vi "Actor Core.vi"(8 "error in":errorcluster, 11 "Configuration in":refnum<class "Configuration.lvclass">) -> (0 "error out":errorcluster, 3 "Actor out":refnum<class "Actor.lvclass">)   [LabVIEW 2016, in "Configuration.lvlib" / "Configuration.lvclass"]
doc: "(<B>Filename</B>: Actor Framework.lvlib:Actor.lvclass:Actor Core.vi)\n\nReceives messages to the actor, reacts to them, and initiates any error handling that may shut the actor down.\n\nDescendant classes may override this VI to append parallel tasks for the actor to complete while it handles messages. Overrides use the Call Parent Method node."
uses:
  <userlib>/Configuration Dialog Actor/Configuration.lvclass
  C:/Program Files (x86)/National Instruments/LabVIEW 2016/vi.lib/ActorFramework/Actor/Actor.lvclass
  <vilib>/ActorFramework/Actor/Actor.lvclass
  <userlib>/Configuration Dialog Actor/Methods/Config Actor Core UI Ref.ctl
  <userlib>/Configuration Dialog Actor/Configuration.lvclass/Configuration.ctl
  <vilib>/ActorFramework/Actor/Actor.lvclass/Actor.ctl
  <vilib>/ActorFramework/Message Enqueuer/Message Enqueuer.lvclass/Message Enqueuer.ctl
  <userlib>/Configuration Dialog Actor/Configuration Messages/Display New Configuration SubPanel Msg/Display New Configuration SubPanel Msg.lvclass/Display New Configuration SubPanel Msg.ctl
  <vilib>/ActorFramework/Message Enqueuer/Init from Existing Queue.vi
  <vilib>/ActorFramework/Message Enqueuer/Enqueue.vi
  <vilib>/ActorFramework/Stop Msg/Stop Msg.lvclass
  C:/Program Files (x86)/National Instruments/LabVIEW 2016/vi.lib/ActorFramework/Message/Message.lvclass
  <userlib>/Configuration Messages/Change Password Msg/Change Password Msg.lvclass
  <userlib>/Configuration Dialog Actor/Configuration Messages/Display New Configuration SubPanel Msg/Display New Configuration SubPanel Msg.lvclass
  <userlib>/Configuration Dialog Actor/Configuration Messages/Display Help for Selected Category Msg/Display Help for Highlighted Category Msg.lvclass
  <vilib>/ActorFramework/Message Priority Queue/Priority Enqueue.vi
  <vilib>/ActorFramework/Message Enqueuer/Message Enqueuer.lvclass
panel:
  in  "Categories":i32(listbox)
  out "Title":string
  in  "Help":bool
  in  "OK":bool
  in  "Cancel":bool
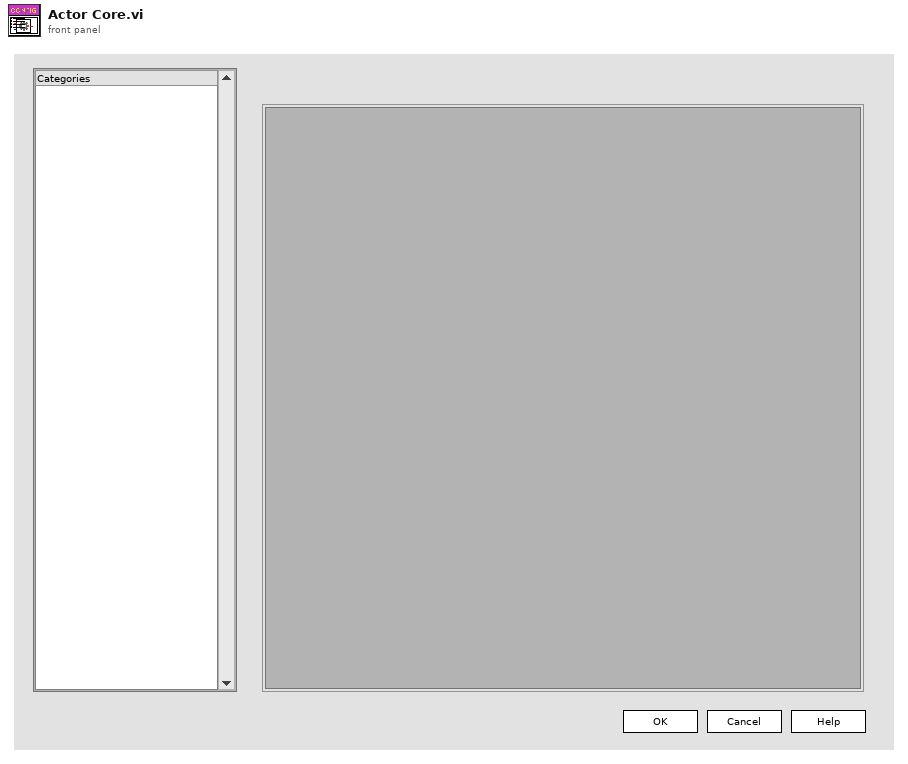
[diagram p1: front panel]
types:
  T1 = typedef "Configuration.lvlib/Configuration.lvclass/Config Actor Core UI Ref.ctl" = cluster{"Title":refnum<vi>, "Sub Panel":refnum<vi>, "OK":refnum<vi>, "Categories":refnum<vi>, "Help":refnum<vi>}
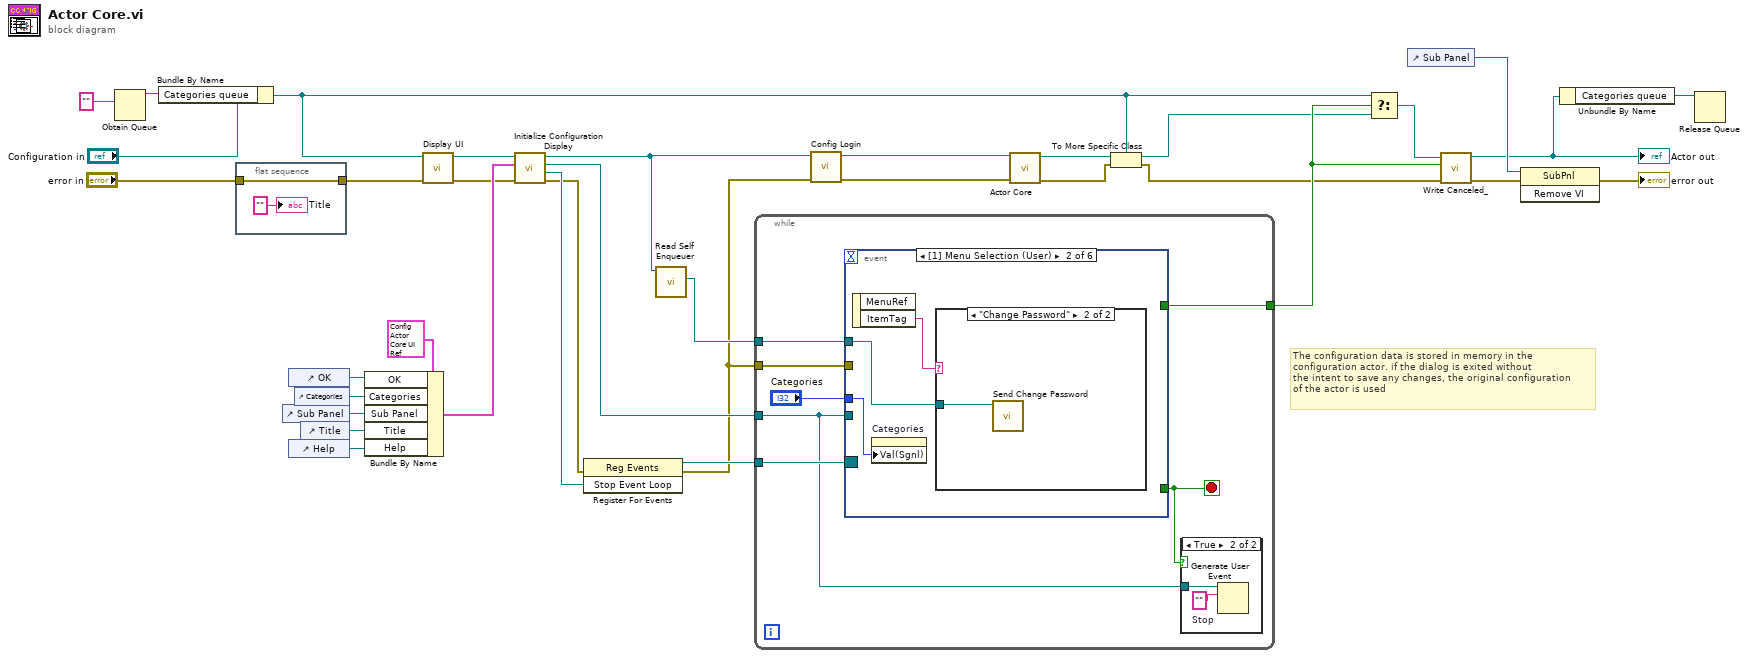
[diagram p0: block diagram]
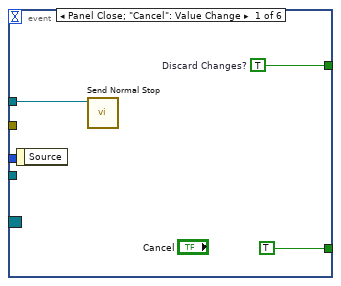
[diagram p3: hidden frame]
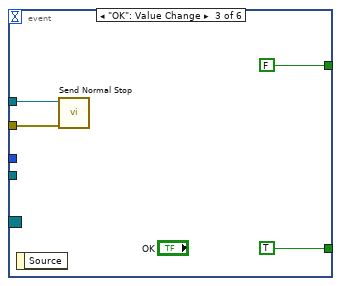
[diagram p5: hidden frame]
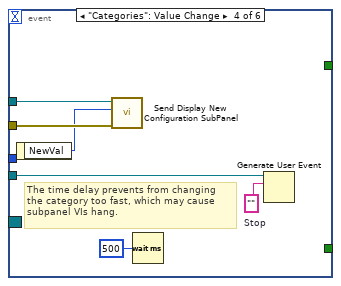
[diagram p6: hidden frame]
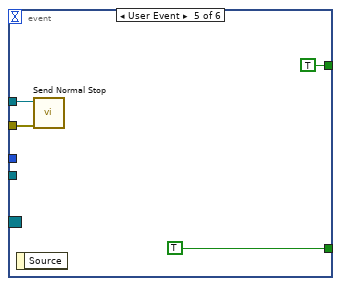
[diagram p7: hidden frame]
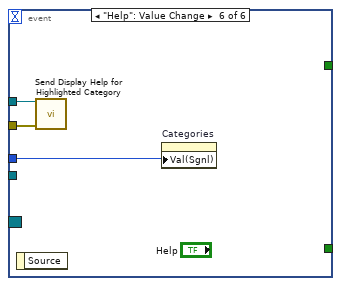
[diagram p8: hidden frame]
diagram:
  # "The configuration data is stored in memory in the\nconfiguration actor. if the dialog is exited without\nthe intent to save any changes, the original configuration\nof the actor is used"
  n1 = Obtain Queue(element data type="") -> (queue out=w4:refnum<queue>)  [unwired: 4 in, 2 out]
  n2 = Bundle By Name(cluster="Configuration in", "Categories queue"=w4) -> (w5:refnum<class "Configuration.lvclass">)
  n3 = flat-sequence {
    tunnel: "error in" -> [w37]
    tunnel: [w37] -> w21
    frame #0 {
      "Title" <- "" ("Title")
    }
  }
  n4 = control-ref of="Sub Panel"() -> (w24:refnum<vi>)
  n5 = control-ref of="OK"() -> (w26:refnum<vi>)
  n6 = control-ref of="Help"() -> (w22:refnum<vi>)
  n7 = control-ref of="Categories"() -> (w25:refnum<vi>)
  n8 = control-ref of="Title"() -> (w23:refnum<vi>)
  n9 = Bundle By Name(cluster=T1 {"Title"=refnum, "Sub Panel"=refnum, "OK"=refnum, "Categories"=refnum, "Help"=refnum} ("Configuration Pane References"), "OK"=w26, "Categories"=w25, "Sub Panel"=w24, "Title"=w23, "Help"=w22) -> (w27:T1)
  n10 = call <userlib>:"Display UI.vi"("error in (no error)"=w21, "Configuration in"=w5) -> ("error out"=w19:errorcluster, "Configuration out"=w20:refnum<class "Configuration.lvclass">)  [unwired: 8 in]
  n11 = call <userlib>:"Initialize Configuration Display.vi"("error in (no error)"=w19, "Configuration Pane References"=w27, "Configuration in"=w20) -> ("error out"=w8:errorcluster, "Stop Event Loop"=w34:refnum<user-event>, "Change Display"=w32:refnum<user-event>, "Configuration out"=w6:refnum<class "Configuration.lvclass">)  [unwired: 5 in]
  n12 = register-events(error in=w8, w34) -> (reference out=w35:refnum<event-registration>, error out=w7:errorcluster)  [unwired: 1 in]
  n13 = call <vilib>:"Read Self Enqueuer.vi"("Actor"=w6) -> ("Self Enqueuer"=w33:refnum<class "Message Enqueuer.lvclass">)  [unwired: 10 in]
  n14 = while {
    tunnel: w35 -> [w44]
    tunnel: w33 -> [w43]
    tunnel: w7 -> [w42]
    tunnel: w32 -> [w39]
    tunnel: [w41] -> w18
    stop <- w40 stop-if-true
    n15 = event shown="[1] Menu Selection (User)" {
      selector: w44 -> [_ _ _ _ _ _]
      dyn-events: _ -> [_ _ _ _ _ _]
      timeout: _ -> [_ _ _ _ _ _]
      tunnel: [TRUE _ TRUE _ TRUE _] -> w40
      tunnel: w43 -> [w49 w51 w56 w62 w65 w70]
      tunnel: w42 -> [_ _ w55 w63 w66 w69]
      tunnel: w39 -> [_ _ _ w58 _ _]
      tunnel: [w47 _ FALSE ("Discard Changes?") _ TRUE ("Discard Changes?") _] -> w41
      tunnel: "Categories" -> [_ w50 _ _ _ w68]
      event Panel Close; "Cancel": Value Change {
        w47 = TRUE  # Discard Changes?
        n16 = event-data() -> ()  [unwired: 1 in, 1 out]
        n17 = call <vilib>:"Send Normal Stop.vi"("Message Enqueuer"=w49) -> ()  [unwired: 10 in, 1 out]
      }
      event Menu Selection (User) {
        n18 = event-data() -> ("ItemTag"=w52:string)  [unwired: 1 in, 1 out]
        n19 = property on="Categories" class="LstBox (strict)"("Val(Sgnl)"=w50) -> ()  [unwired: 2 in, 2 out]
        n20 = case shown="\"Change Password\"" w52 {
          tunnel: w51 -> [_ w53]
          frame Default {
          }
          frame "Change Password" {
            n21 = call <userlib>:"Send Change Password.vi"("Message Enqueuer"=w53) -> ()  [unwired: 9 in, 2 out]
          }
        }
      }
      event "OK": Value Change {
        n22 = event-data() -> ()  [unwired: 1 in, 1 out]
        n23 = call <vilib>:"Send Normal Stop.vi"("error in (no error)"=w55, "Message Enqueuer"=w56) -> ()  [unwired: 9 in, 1 out]
      }
      event "Categories": Value Change {
        w59 = ""  # Stop
        # "The time delay prevents from changing\nthe category too fast, which may cause\nsubpanel VIs hang."
        n24 = event-data() -> ("NewVal"=w61:i32)  [unwired: 1 in]
        n25 = call <userlib>:"Send Display New Configuration SubPanel.vi"("error in (no error)"=w63, "ListBox Selection"=w61, "Message Enqueuer"=w62) -> ()  [unwired: 7 in, 2 out]
        n26 = Wait (ms)(milliseconds to wait=u32 500) -> ()  [unwired: 1 out]
        n27 = Generate User Event(user event=w58, event data cluster=w59) -> ()  [unwired: 2 in, 2 out]
      }
      event User Event {
        n28 = event-data() -> ()  [unwired: 1 in, 1 out]
        n29 = call <vilib>:"Send Normal Stop.vi"("error in (no error)"=w66, "Message Enqueuer"=w65) -> ()  [unwired: 9 in, 1 out]
      }
      event "Help": Value Change {
        n30 = event-data() -> ()  [unwired: 1 in, 1 out]
        n31 = call <userlib>:"Send Display Help for Highlighted Category.vi"("error in (no error)"=w69, "Message Enqueuer"=w70) -> ()  [unwired: 8 in, 2 out]
        n32 = property on="Categories" class="LstBox (strict)"("Val(Sgnl)"=w68) -> ()  [unwired: 2 in, 2 out]
      }
    }
    n33 = case shown="True" w40 {
      tunnel: w39 -> [_ w45]
      frame False {
      }
      frame True {
        w46 = ""  # Stop
        n34 = Generate User Event(user event=w45, event data cluster=w46) -> ()  [unwired: 2 in, 2 out]
      }
    }
  }
  n35 = call <userlib>:"Config Login.vi"("error in (no error)"=w7, "Configuration in"=w6) -> ("error out"=w9:errorcluster, "Configuration out"=w10:refnum<class "Configuration.lvclass">)  [unwired: 8 in]
  n36 = call-parent "Actor Core.vi"("error in"=w9, "Actor in"=w10) -> ("error out"=w14:errorcluster, "Actor out"=w16:refnum<class "Actor.lvclass">)  [unwired: 8 in]
  n37 = To More Specific Class(target class=w5, reference=w16, error in=w14) -> (specific class reference=w15:refnum<class "Configuration.lvclass">, error out=w13:errorcluster)
  n38 = Select(t=w5, s=w18, f=w15) -> (s? t:f=w12:refnum<class "Configuration.lvclass">)
  n39 = control-ref of="Sub Panel"() -> (w30:refnum<vi>)
  n40 = call <userlib>:"Write Canceled_.vi"("error in (no error)"=w13, "Canceled?"=w18, "Configuration in"=w12) -> ("error out"=w17:errorcluster, "Configuration out"=w2:refnum<class "Configuration.lvclass">)  [unwired: 7 in]
  "Actor out" <- w2
  n41 = invoke class="SubPnl" method="Remove VI"(reference=w30, error in=w17) -> (error out=→"error out":errorcluster)  [unwired: 1 in, 2 out]
  n42 = Unbundle By Name(w2) -> ("Categories queue"=w1:refnum<queue>)
  n43 = Release Queue(queue=w1) -> ()  [unwired: 2 in, 3 out]
